vi "接口报文存储.vi"(4 "IP-Port":string, 5 "动作":string(combo), 6 "客服端键":string, 8 "error in (no error)":errorcluster caption="错误输入（无错误）", 10 "报文":string, 11 "MainPage 输入":refnum<class "MainPage.lvclass">) -> (0 "error out":errorcluster caption="错误输出", 2 "报文输出":string, 3 "MainPage 输出":refnum<class "MainPage.lvclass">)   [LabVIEW 2019, in "MainPage.lvlib" / "MainPage.lvclass"]
uses:
  MainPage.lvclass
panel:
  in  "接口正常？":bool
  # "未使用"
  # "接口错误时报文为空"
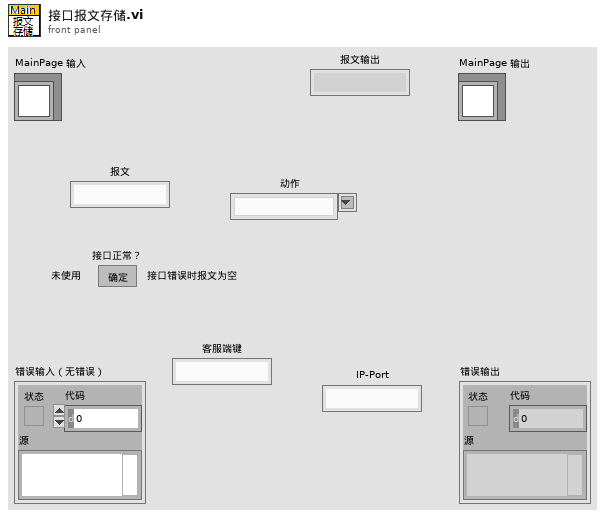
[diagram p1: front panel]
types:
  T1 = cluster{"寄存器模拟":u16[], "串口正常？":bool, "报文信息记录":string[][]}
  T2 = enum16{"ini", "增加记录", "读取记录", "更改寄存器值", "更改接口状态", "更改报文信息", "增加报文信息"}
  T3 = cluster{"串口正常？":bool, "寄存器模拟":u16[], "报文信息记录":string[][]}
  T4 = enum16{"ini", "读取", "写入-报文记录", "写入-寄存器模拟", "写入-串口状态", "增加报文记录"}
  T5 = typedef "MainPage.lvlib/MainPage.lvclass/DataRef_通讯接口.ctl" = cluster{"连接方式":enum16{"网口(客服端)", "网口(服务端)", "串口"}, "VISA串口名称":refnum<visa-resource-name>, "服务端识别":cluster{"本机IP":string, "本机端口":u16, "当前目标":string, "服务端侦听ID":refnum<k5>}, "客服端识别":cluster{"客P-主IP:Port":string}, "客服端记录":map{string, refnum<k5>}, "服务端接口记录":map{string, refnum<k5>}}
  T6 = typedef "MainPage.lvlib/MainPage.lvclass/通用配置选项.ctl" = cluster{"ModBusRTU反馈":enum32{"模拟反馈", "无反馈", "错误反馈"}, "侦听周期":u32, "跳转反馈":bool, "报文记录数量":u16, "客服端新增模式":enum32{"单端模式", "多端共存"}}
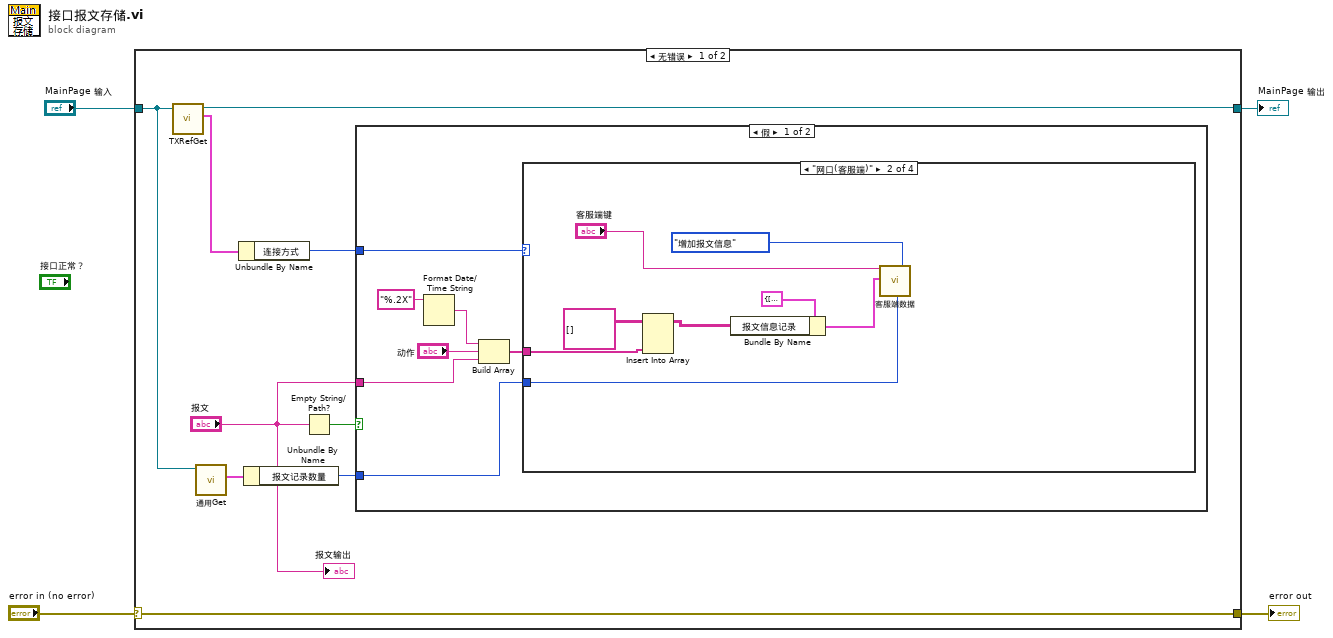
[diagram p0: block diagram]
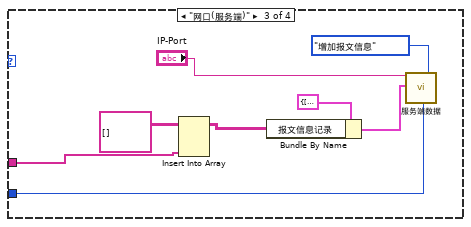
[diagram p3: hidden frame]
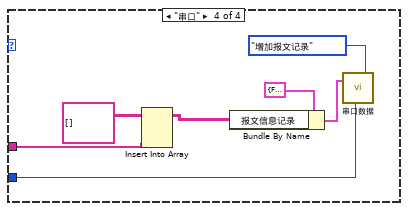
[diagram p4: hidden frame]
diagram:
  n1 = case shown="无错误" "error in (no error)" {
    selector: "error in (no error)" -> [w13 w45]
    tunnel: [w13 w45] -> w3
    tunnel: [w5 w44] -> w1
    tunnel: "MainPage 输入" -> [w8 w44]
    frame No Error {
      n2 = call-dynamic "TXRefGet.vi"("MainPage 输入"=w8) -> ("通讯接口数据"=w12:T5, "MainPage 输出"=w5:refnum<class "MainPage.lvclass">)  [unwired: 6 in, 3 out]
      n3 = call-dynamic "通用Get.vi"("MainPage 输入"=w8) -> ("通用配置"=w7:T6)  [unwired: 6 in, 4 out]
      n4 = Unbundle By Name(w12) -> ("连接方式"=w11:enum16{"网口(客服端)", "网口(服务端)", "串口"})
      n5 = Unbundle By Name(w7) -> ("报文记录数量"=w6:u16)
      n6 = Empty String/Path?(string/path="报文") -> (empty?=w10:bool)
      n7 = case shown="假" w10 {
        tunnel: w11 -> [w20 _]
        tunnel: "报文" -> [w17 _]
        tunnel: w6 -> [w14 _]
        frame False {
          n8 = Format Date/Time String(time format string (%c)="%.2X" ("时间格式字符串(%c)")) -> (date/time string=w18:string)  [unwired: 2 in]
          n9 = Build Array(w18, "动作", w17) -> (w15:string[])
          n10 = case shown="\"网口(客服端)\"" w20 {
            tunnel: w15 -> [_ w24 w30 w39]
            tunnel: w14 -> [_ w27 w34 w43]
            frame Default {
            }
            frame "网口(客服端)" {
              n11 = Insert Into Array(array=string[][] [], new element=w24) -> (w21:string[][])  [unwired: 2 in]
              n12 = Bundle By Name(cluster=T1 {"寄存器模拟"=[], "串口正常？"=FALSE, "报文信息记录"=[]} ("数据输入"), "报文信息记录"=w21) -> (w22:T1)
              n13 = call "客服端数据.vi"("客P-主IP:P"="客服端键", "数据输入"=w22, "报文最大量"=w27, "枚举"=T2."增加报文信息") -> ()  [unwired: 14 in, 2 out]
            }
            frame "网口(服务端)" {
              n14 = Insert Into Array(array=string[][] [], new element=w30) -> (w31:string[][])  [unwired: 2 in]
              n15 = Bundle By Name(cluster=T1 {"寄存器模拟"=[], "串口正常？"=FALSE, "报文信息记录"=[]} ("数据输入"), "报文信息记录"=w31) -> (w29:T1)
              n16 = call "服务端数据.vi"("IP-Port"="IP-Port", "数据输入"=w29, "报文最大量"=w34, "枚举"=T2."增加报文信息") -> ()  [unwired: 14 in, 2 out]
            }
            frame "串口" {
              n17 = Insert Into Array(array=string[][] [], new element=w39) -> (w40:string[][])  [unwired: 2 in]
              n18 = Bundle By Name(cluster=T3 {"串口正常？"=FALSE, "寄存器模拟"=[], "报文信息记录"=[]} ("串口输入"), "报文信息记录"=w40) -> (w37:T3)
              n19 = call "串口数据.vi"("串口输入"=w37, "报文最大值"=w43, "枚举"=T4."增加报文记录") -> ()  [unwired: 16 in, 1 out]
            }
          }
        }
        frame True {
        }
      }
      "报文输出" <- "报文"
    }
    frame Error {
    }
  }
  "error out" <- w3
  "MainPage 输出" <- w1
